vi "Calculate High-Low time.vi"(11 "Status":T1 {"Setting"."X Pos." scale=-2.0..2.0; "Setting"."Y Pos." scale=-2.0..2.0}) -> (2 "low time":dbl, 3 "high time":dbl)   [LabVIEW 2013]
uses:
  init & communication/init-status.ctl
  init & communication/Setting.ctl
  init & communication/event-package.ctl
  init & communication/Event1.ctl
  init & communication/data-package.ctl
  init & communication/Event.ctl
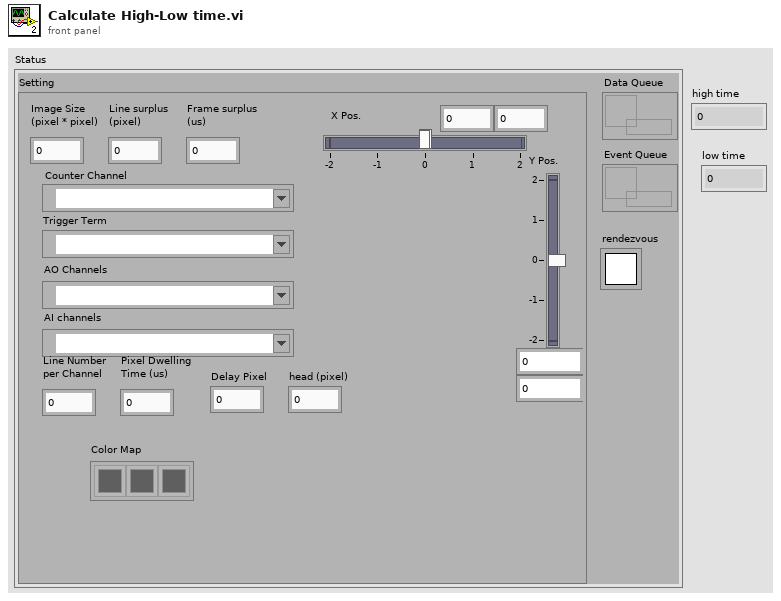
[diagram p1: front panel]
types:
  T1 = typedef "init-status.ctl" = cluster{"Setting":T2, "Event Queue":refnum<queue>, "Data Queue":refnum<queue>, "rendezvous":T3}
  T2 = typedef "Setting.ctl" = cluster{"Image Size\n(pixel * pixel)":i32, "Counter Channel":tag, "Trigger Term":tag, "AO Channels":tag, "Y Pos.":cluster{dbl, dbl}, "X Pos.":cluster{dbl, dbl}, "Line surplus\n(pixel)":i32, "Frame surplus\n(us)":i32, "AI channels":tag, "Line Number\nper Channel":i32, "Delay Pixel":i32, "Pixel Dwelling\nTime (us)":i32, "Color Map":u32[], "head (pixel)":i32}
  T3 = typedef "Rendezvous RefNum" = refnum<k1>
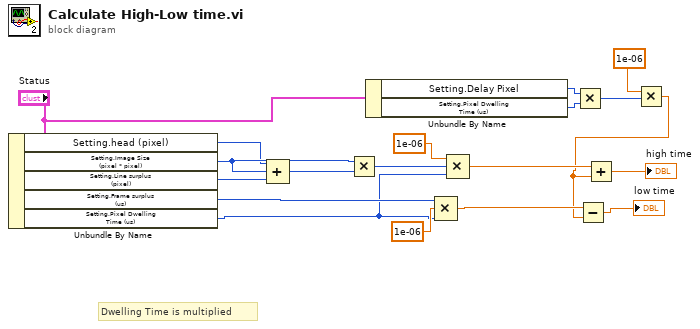
[diagram p0: block diagram]
diagram:
  # "Dwelling Time is multiplied"
  n1 = Unbundle By Name("Status") -> ("Setting.head (pixel)"=w1:i32, "Setting.Image Size\n(pixel * pixel)"=w17:i32, "Setting.Line surplus\n(pixel)"=w19:i32, "Setting.Frame surplus\n(us)"=w13:i32, "Setting.Pixel Dwelling\nTime (us)"=w12:i32)
  n2 = Compound Arithmetic op=ADD(w1, w17, w19) -> (w18:i32)
  n3 = Multiply(x=w17, y=w18) -> (x*y=w16:i32)
  n4 = Unbundle By Name("Status") -> ("Setting.Delay Pixel"=w10:i32, "Setting.Pixel Dwelling\nTime (us)"=w9:i32)
  n5 = Compound Arithmetic op=MULTIPLY(w13, 1e-06 ("x"), w12) -> (w6:dbl)
  n6 = Compound Arithmetic op=MULTIPLY(1e-06 ("x"), w16, w12) -> (w8:dbl)
  n7 = Multiply(x=w10, y=w9) -> (x*y=w4:i32)
  n8 = Multiply(x=1e-06, y=w4) -> (x*y=w2:dbl)
  n9 = Subtract(x=w6, y=w2) -> (x-y=→"low time":dbl)
  n10 = Add(x=w8, y=w2) -> (x+y=→"high time":dbl)
